vi "New from bytes.vi"(8 "error in (no error)":errorcluster, 11 "bytes":u8[](array[numeric])) -> (0 "error out":errorcluster, 1 "Timestamp":timestamp, 2 "MsgPackTimestamp out":refnum<class "MsgPackTimestamp.lvclass">, 3 "remaining bytes":u8[](array[numeric]))   [LabVIEW 2020, in "MessagePack.lvlib" / "MsgPackTimestamp.lvclass"]
uses:
  MsgPackTimestamp.lvclass
  C:/local/wamplv/MessagePack/MsgPackExt/MsgPackExt.lvclass
  MsgPackExt/MsgPackExt.lvclass/MsgPackExt.ctl
  MsgPackTimestamp.lvclass/MsgPackTimestamp.ctl
  MsgPackExt/Accessors/Read Payload Ext Type.vi
  Private/Raise bad data error.vi
  <vilib>/Utility/error.llb/Error Cluster From Error Code.vi
  <vilib>/LabVIEW Open Source Project/Epoch Date & Time/epoch.UNIX/Epoch.UNIX.lvclass
  MsgPackExt/MsgPackExt.lvclass
  MessagePack.lvlib
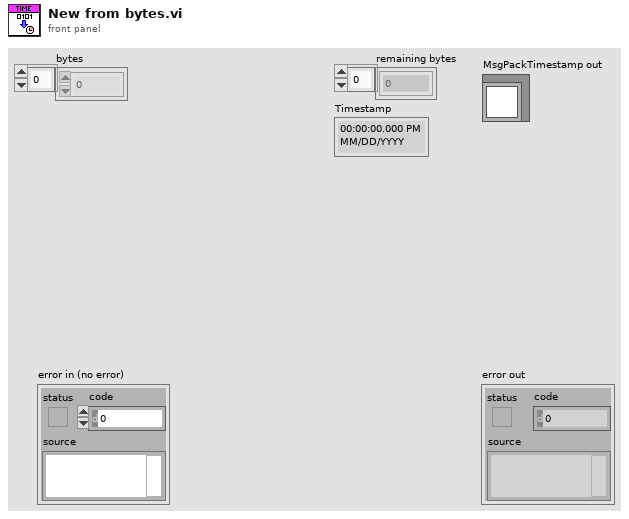
[diagram p1: front panel]
types:
  T1 = typedef "MessagePack.lvlib/MsgPack Object Types.ctl" = enum16{"UNSUPPORTED", "POSINT", "NEGINT", "FIXMAP", "FIXARRAY", "FIXSTR", "NIL", "FALSE", "TRUE", "BIN8", "BIN16", "BIN32", "EXT8", "EXT16", "EXT32", "FLOAT32", "FLOAT64", "UINT8", "UINT16", "UINT32", "UINT64", "INT8", "INT16", "INT32", "INT64", "FIXEXT1", "FIXEXT2", "FIXEXT4", "FIXEXT8", "FIXEXT16", "STR8", "STR16", "STR32", "ARRAY16", "ARRAY32", "MAP16", "MAP32"}
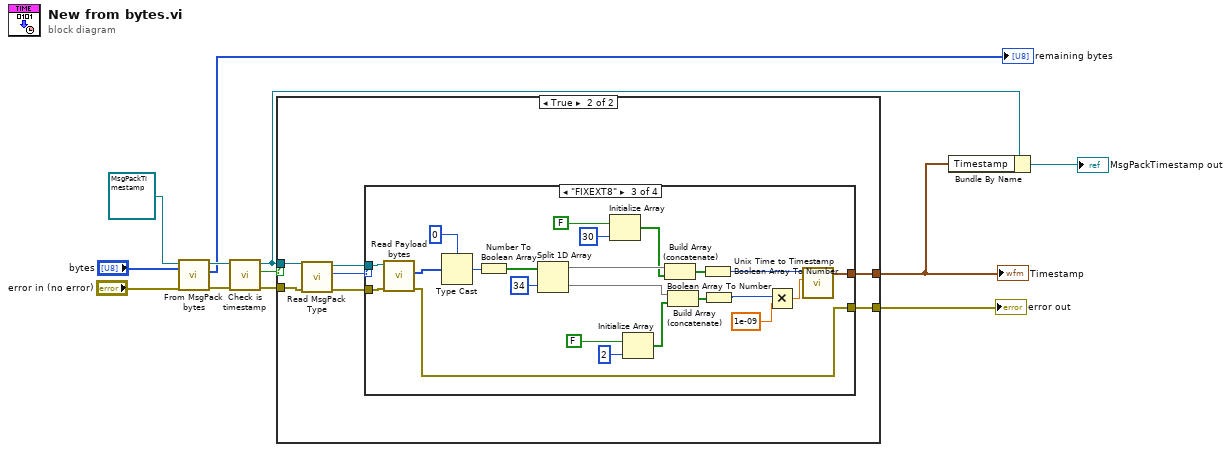
[diagram p0: block diagram]
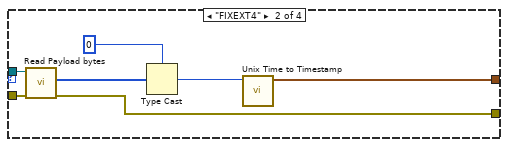
[diagram p4: hidden frame]
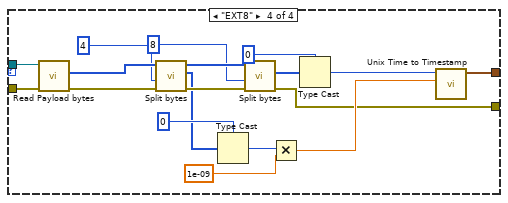
[diagram p5: hidden frame]
diagram:
  n1 = call-dynamic "From MsgPack bytes.vi"("error in (no error)"="error in (no error)", "Bytes in"="bytes", "MessagePack.lvlib:MsgPackExt.lvclass"=refnum<class "MsgPackTimestamp.lvclass"> refnum ("MessagePack.lvlib:MsgPackTimestamp.lvclass")) -> ("error out"=w9:errorcluster, "remaining bytes"=→"remaining bytes":u8[], "MsgPackExt"=w8:refnum<class "MsgPackTimestamp.lvclass">)  [unwired: 6 in]
  n2 = call "Check is timestamp.vi"("error in (no error)"=w9, "MessagePack.lvlib:MsgPackTimestamp.lvclass"=w8) -> ("error out"=w7:errorcluster, "Valid?"=w6:bool, "MessagePack.lvlib:MsgPackTimestamp.lvclass 2"=w4:refnum<class "MsgPackTimestamp.lvclass">)  [unwired: 7 in]
  n3 = case shown="True" w6 {
    tunnel: w7 -> [w13 w20]
    tunnel: w4 -> [_ w19]
    tunnel: [_ w15] -> w2
    tunnel: [w13 w14] -> w1
    frame False {
    }
    frame True {
      n4 = call "Read MsgPack Type.vi"("error in (no error)"=w20, "MsgPackExt in"=w19) -> ("error out"=w17:errorcluster, "MsgPack Object Type"=w18:T1, "MsgPackExt out"=w16:refnum<class "MsgPackTimestamp.lvclass">)  [unwired: 7 in]
      n5 = case shown="\"FIXEXT8\"" w18 {
        tunnel: w17 -> [w21 w28 w31 w69]
        tunnel: w16 -> [_ w27 w30 w68]
        tunnel: [_ w23 w33 w53] -> w15
        tunnel: [w21 w22 w32 w52] -> w14
        frame "UNSUPPORTED", Default {
        }
        frame "FIXEXT4" {
          n6 = call "Read Payload bytes.vi"("error in (no error)"=w28, "MsgPackExt in"=w27) -> ("error out"=w22:errorcluster, "Payload bytes"=w26:u8[])  [unwired: 7 in, 1 out]
          n7 = Type Cast(type=u32 0, x=w26) -> (*(type *) &x=w24:u32)
          n8 = call <vilib>:"Unix Time to Timestamp.vi"("Unix Time (s)"=w24) -> ("Timestamp"=w23:timestamp)  [unwired: 9 in, 1 out]
        }
        frame "FIXEXT8" {
          n9 = call "Read Payload bytes.vi"("error in (no error)"=w31, "MsgPackExt in"=w30) -> ("error out"=w32:errorcluster, "Payload bytes"=w29:u8[])  [unwired: 7 in, 1 out]
          n10 = Type Cast(type=u64 0, x=w29) -> (*(type *) &x=w50:u64)
          n11 = Number To Boolean Array(number=w50) -> (Boolean array=w49:bool[])
          n12 = Split 1D Array(array=w49, index=34) -> (first subarray=w46:bool[], second subarray=w39:bool[])
          n13 = Initialize Array(FALSE, 30 ("dimension size")) -> (w44:bool[])
          n14 = Initialize Array(FALSE, 2 ("dimension size")) -> (w38:bool[])
          n15 = Build Array (concatenate)(w46, w44) -> (w40:bool[])
          n16 = Build Array (concatenate)(w39, w38) -> (w37:bool[])
          n17 = Boolean Array To Number(Boolean array=w40) -> (number=w43:u64)
          n18 = Boolean Array To Number(Boolean array=w37) -> (number=w35:u32)
          n19 = Multiply(x=w35, y=1e-09) -> (x*y=w34:dbl)
          n20 = call <vilib>:"Unix Time to Timestamp.vi"("Fractional Second"=w34, "Unix Time (s)"=w43) -> ("Timestamp"=w33:timestamp)  [unwired: 8 in, 1 out]
        }
        frame "EXT8" {
          n21 = call "Read Payload bytes.vi"("error in (no error)"=w69, "MsgPackExt in"=w68) -> ("error out"=w66:errorcluster, "Payload bytes"=w67:u8[])  [unwired: 7 in, 1 out]
          n22 = call "Split bytes.vi"("error in"=w66, "count (1)"=4, "bytes in"=w67) -> ("error out"=w65:errorcluster, "selected bytes"=w61:u8[], "remaining bytes"=w64:u8[])  [unwired: 5 in, 1 out]
          n23 = Type Cast(type=u32 0, x=w61) -> (*(type *) &x=w56:u32)
          n24 = call "Split bytes.vi"("error in"=w65, "count (1)"=8, "bytes in"=w64) -> ("error out"=w52:errorcluster, "selected bytes"=w58:u8[])  [unwired: 5 in, 2 out]
          n25 = Multiply(x=w56, y=1e-09) -> (x*y=w54:dbl)
          n26 = Type Cast(type=i64 0, x=w58) -> (*(type *) &x=w57:i64)
          n27 = call <vilib>:"Unix Time to Timestamp.vi"("Fractional Second"=w54, "Unix Time (s)"=w57) -> ("Timestamp"=w53:timestamp)  [unwired: 8 in, 1 out]
        }
      }
    }
  }
  "error out" <- w1
  "Timestamp" <- w2
  n28 = Bundle By Name(cluster=w4, "Timestamp"=w2) -> (→"MsgPackTimestamp out":refnum<class "MsgPackTimestamp.lvclass">)
